vi "SWERVE_DRIVE_MODULE_ACT.vi"(8 "SwervePosInDeadband":bool=TRUE, 9 "Swerve Sense":T2={"Speed"=0.0, "Angle"={"VALUE"=0.0, "COS"=1.0, "SIN"=0.0}} {"Angle"."SIN" format="%13.4f"; "Angle"."COS" format="%13.4f"; "Angle"."VALUE" format="%13.4f"}, 10 "Swerve Dmd":T2={"Speed"=0.0, "Angle"={"VALUE"=0.0, "COS"=1.0, "SIN"=0.0}} {"Angle"."SIN" format="%13.4f"; "Angle"."COS" format="%13.4f"; "Angle"."VALUE" format="%13.4f"}, 11 "Swerve Module TypDef":T4) -> (0 "SwerveOnTarget":bool, 1 "SwervePosError":dbl, 2 "Swerve Motor Dmd":dbl, 3 "Wheel Motor Dmd":dbl, 4 "WheelSpeedErr":dbl)   [LabVIEW 2019]
uses:
  SWERVE_DRIVE_MODULE_TYPDEF.ctl
  <vilib>/Rock Robotics/WPI/MotorControl/WPI_MotorControlDeviceRef.ctl
  <vilib>/Rock Robotics/WPI/MotorControl/WPI_MotorControlType.ctl
  <vilib>/Rock Robotics/SystemInterfaces/DIO/FPGA_DIOPWMChannel.ctl
  <vilib>/Rock Robotics/WPI/PWM/WPI_PWMDeadband.ctl
  <vilib>/Rock Robotics/SystemInterfaces/DIO/FPGA_DIOChannel.ctl
  <vilib>/Rock Robotics/WPI/Encoder/WPI_EncoderDevRef.ctl
  <vilib>/Rock Robotics/SystemInterfaces/Encoder/FPGA_EncoderIdx.ctl
  <vilib>/Rock Robotics/SystemInterfaces/Counter/FPGA_CounterCtrSystemIndex.ctl
  <vilib>/Rock Robotics/WPI/Encoder/WPI_EncoderType.ctl
  <vilib>/Rock Robotics/WPI/ThirdParty/JAS_Junk/TrajLib/TypeDef/SWERVE_DRIVE_MODULE_STATE.ctl
  <vilib>/Rock Robotics/WPI/ThirdParty/JAS_Junk/TrajLib/TypeDef/ROTATION2D.ctl
  SWERVE_MODULE_MOTOR_CO.ctl
  <vilib>/Rock Robotics/WPI/ThirdParty/JAS_Junk/TrajLib/SlewRateLimiter_New.vi
  <vilib>/Rock Robotics/WPI/ThirdParty/JAS_Junk/TrajLib/SlewRateLimiter_Reset.vi
  <vilib>/Rock Robotics/WPI/ThirdParty/JAS_Junk/TrajLib/SlewRateLimiter_Calculate.vi
  <vilib>/Rock Robotics/WPI/ThirdParty/JAS_Junk/TrajLib/SlewRateLimiter_SetRate.vi
  <vilib>/Rock Robotics/WPI/ThirdParty/JAS_Junk/TrajLib/Util_GetTime.vi
  <vilib>/addons/control/pid/pid.llb/PID (DBL).vi
  <vilib>/addons/control/pid/NI_PID_pid.lvlib
  Secret_Control_Library_Protected/Secret_Control_Library_Protected.lvlib
  <vilib>/Rock Robotics/WPI/ThirdParty/JAS_Junk/TrajLib/Trajectory_Library.lvlib
panel:
  in  "Speed PID":T1={"proportional gain (Kc)"=0.45, "integral time (Ti, min)"=0.008, "derivative time (Td, min)"=0.0} {"derivative time (Td, min)" format="%.3f"; "integral time (Ti, min)" format="%.3f"; "proportional gain (Kc)" format="%.3f"}
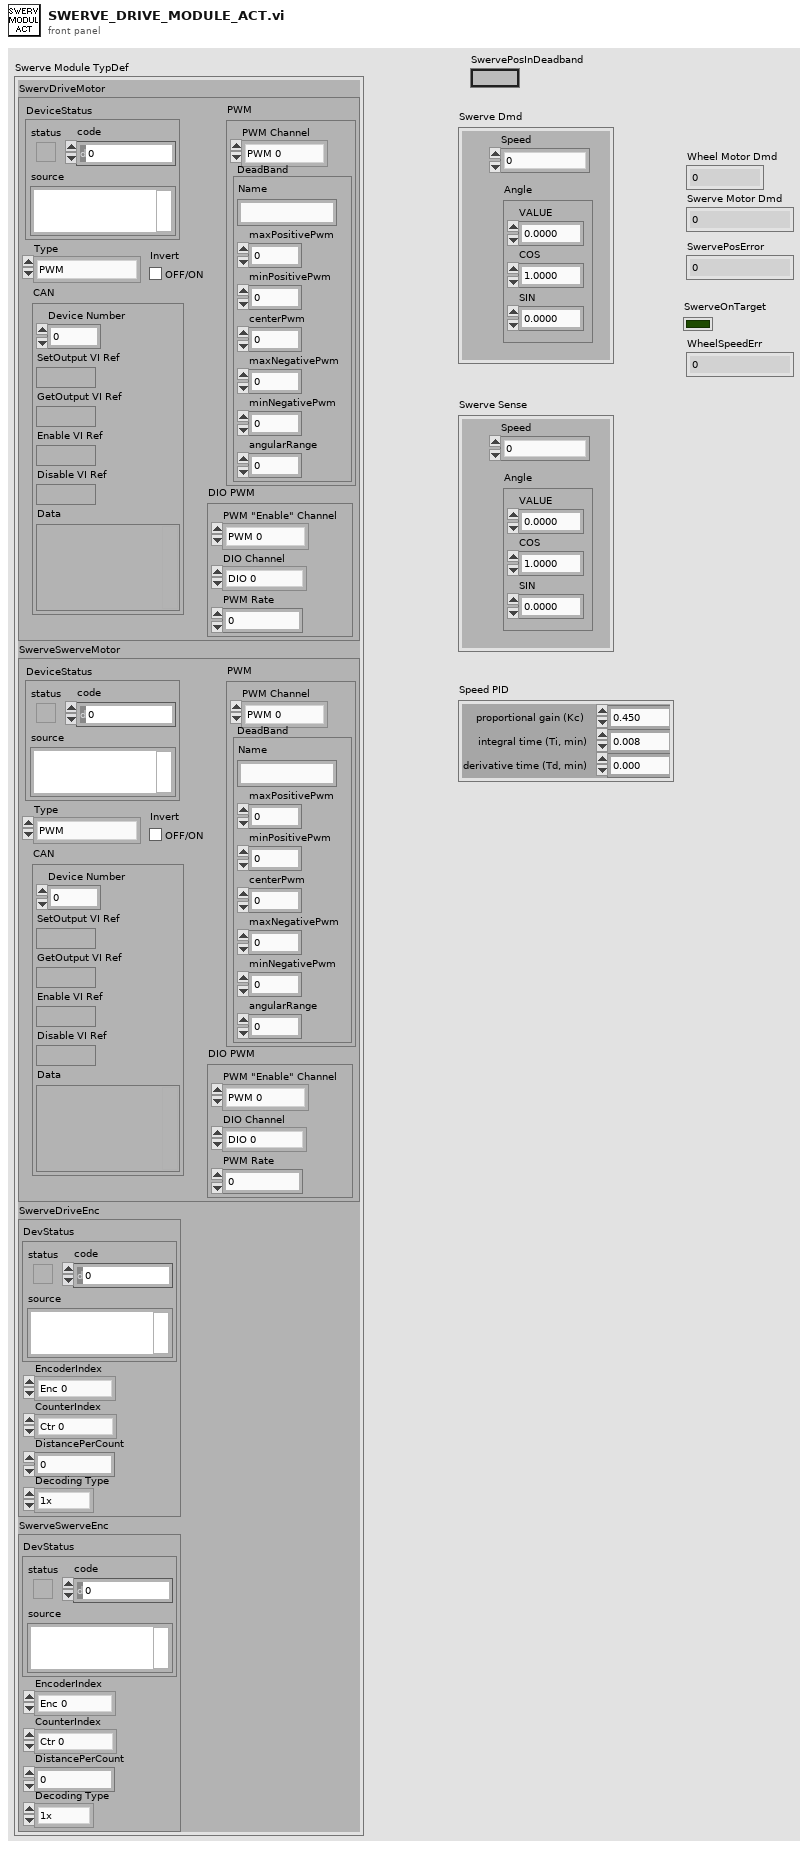
[diagram p1: front panel]
types:
  T1 = cluster{"proportional gain (Kc)":dbl, "integral time (Ti, min)":dbl, "derivative time (Td, min)":dbl}
  T2 = typedef "Trajectory_Library.lvlib/SWERVE_DRIVE_MODULE_STATE.ctl" = cluster{"Speed":dbl, "Angle":T3}
  T3 = typedef "Trajectory_Library.lvlib/ROTATION2D.ctl" = cluster{"VALUE":dbl, "COS":dbl, "SIN":dbl}
  T4 = typedef "SWERVE_DRIVE_MODULE_TYPDEF.ctl" = cluster{"SwervDriveMotor":T5, "SwerveSwerveMotor":T5, "SwerveDriveEnc":T10, "SwerveSwerveEnc":T10}
  T5 = typedef "WPI_MotorControlDeviceRef.ctl" = cluster{"DeviceStatus":errorcluster, "Type":T6, "PWM":cluster{"PWM Channel":T7, "DeadBand":T8}, "CAN":cluster{"Device Number":u8, "SetOutput VI Ref":variant, "GetOutput VI Ref":variant, "Enable VI Ref":variant, "Disable VI Ref":variant, "Data":variant}, "Invert":bool, "DIO PWM":cluster{"PWM \"Enable\" Channel":T7, "DIOChannel":T9, "PWM Rate":dbl}}
  T6 = typedef "WPI_MotorControlType.ctl" = enum16{"PWM", "CAN", "DIO PWM"}
  T7 = typedef "FPGA_DIOPWMChannel.ctl" = enum8{"PWM 0", "PWM 1", "PWM 2", "PWM 3", "PWM 4", "PWM 5", "PWM 6", "PWM 7", "PWM 8", "PWM 9", "PWM MXP 0", "PWM MXP 1", "PWM MXP 2", "PWM MXP 3", "PWM MXP 4", "PWM MXP 5", "PWM MXP 6", "PWM MXP 7", "PWM MXP 8", "PWM MXP 9", "Invalid"}
  T8 = typedef "WPI_PWMDeadband.ctl" = cluster{"Name":string, "maxPositivePwm":i32, "minPositivePwm":i32, "centerPwm":i32, "maxNegativePwm":i32, "minNegativePwm":i32, "angularRange":u16}
  T9 = typedef "FPGA_DIOChannel.ctl" = enum8{"DIO 0", "DIO 1", "DIO 2", "DIO 3", "DIO 4", "DIO 5", "DIO 6", "DIO 7", "DIO 8", "DIO 9", "DIO MXP 0", "DIO MXP 1", "DIO MXP 2", "DIO MXP 3", "DIO MXP 4", "DIO MXP 5", "DIO MXP 6", "DIO MXP 7", "DIO MXP 8", "DIO MXP 9", "DIO MXP 10", "DIO MXP 11", "DIO MXP 12", "DIO MXP 13", "DIO MXP 14", "DIO MXP 15", "SPI Port CS1", "SPI Port CS2", "SPI Port CS3", "SPI Port MISO", "SPI Port MOSI", "Invalid"}
  T10 = typedef "WPI_EncoderDevRef.ctl" = cluster{"DevStatus":errorcluster, "EncoderIndex":T11, "CounterIndex":T12, "DistancePerCount":dbl, "Decoding Type":T13}
  T11 = typedef "FPGA_EncoderIdx.ctl" = enum8{"Enc 0", "Enc 1", "Enc 2", "Enc 3", "Enc 4", "Enc 5", "Enc 6", "Enc 7", "Invalid"}
  T12 = typedef "FPGA_CounterCtrSystemIndex.ctl" = enum8{"Ctr 0", "Ctr 1", "Ctr 2", "Ctr 3", "Ctr 4", "Ctr 5", "Ctr 6", "Ctr 7", "Invalid"}
  T13 = typedef "WPI_EncoderType.ctl" = enum16{"1x", "2x", "4x"}
  T14 = typedef "SWERVE_MODULE_MOTOR_CO.ctl" = cluster{"WheelMotorDmd":dbl, "SwerveMotorDmd":dbl}
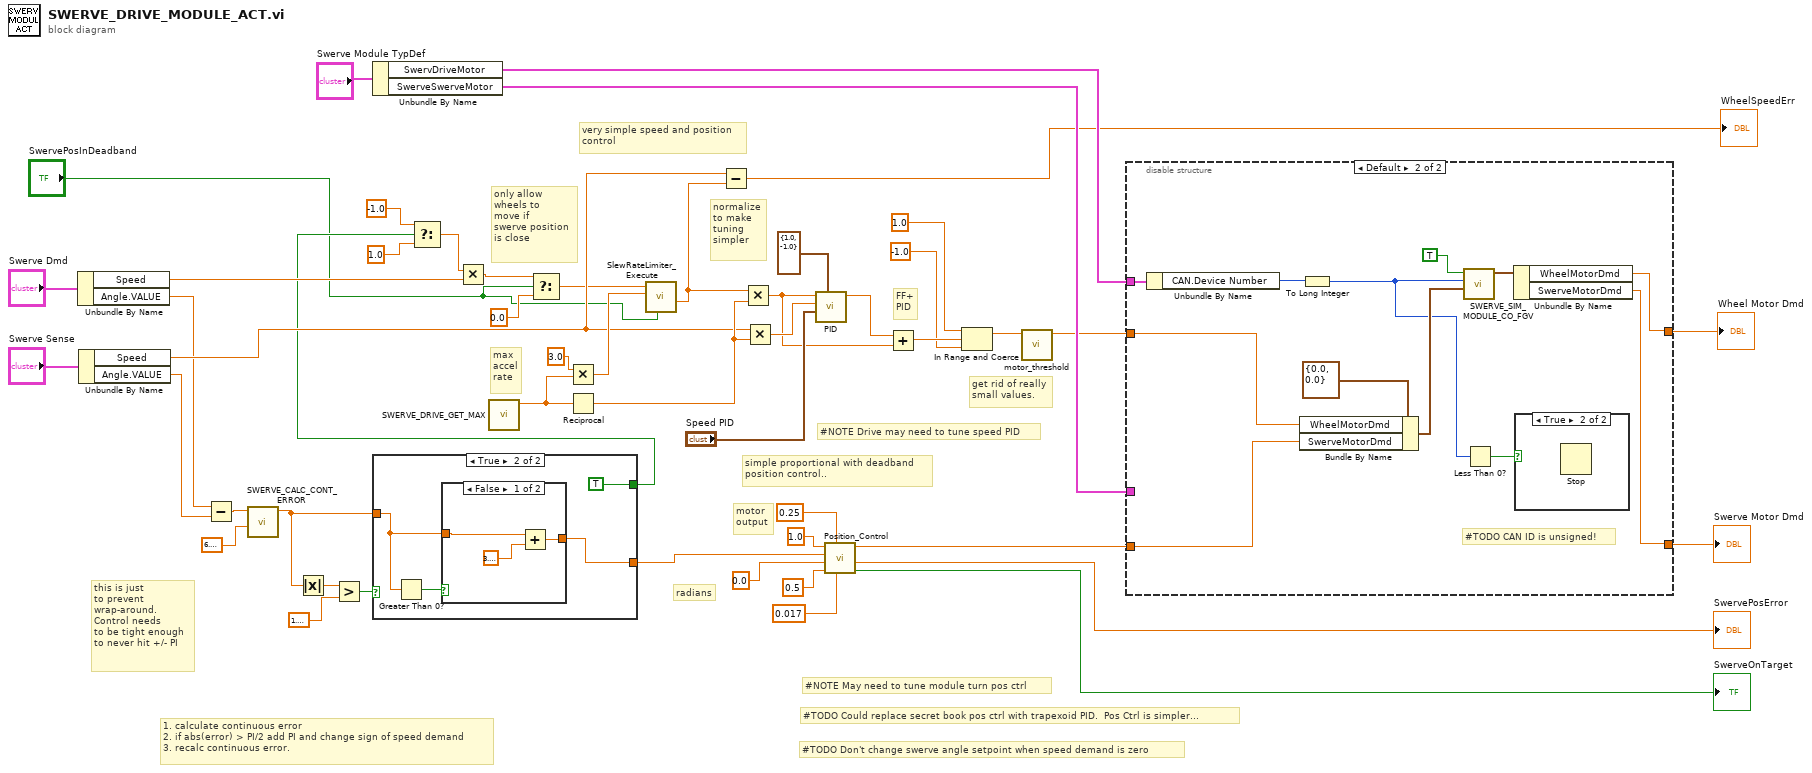
[diagram p0: block diagram]
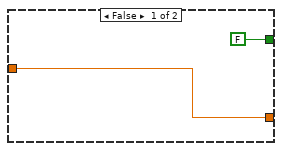
[diagram p2: hidden frame]
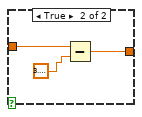
[diagram p3: hidden frame]
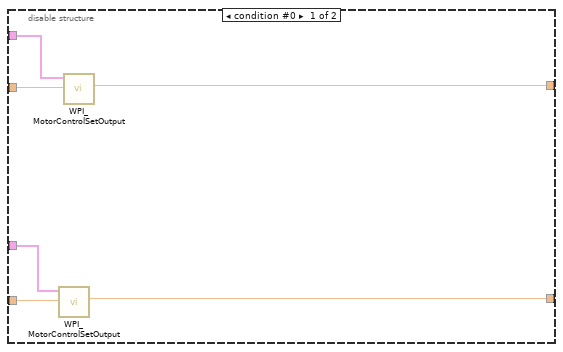
[diagram p4: hidden frame]
diagram:
  # "only allow\nwheels to \nmove if \nswerve position\nis close"
  # "#TODO Don't change swerve angle setpoint when speed demand is zero"
  # "1. calculate continuous error\n2. if abs(error) > PI/2 add PI and change sign of speed demand\n3. recalc continuous error."
  # "radians"
  # "#NOTE Drive may need to tune speed PID"
  # "#TODO Could replace secret book pos ctrl with trapexoid PID.  Pos Ctrl is simpler..."
  # "#NOTE May need to tune module turn pos ctrl"
  # "simple proportional with deadband\nposition control.."
  # "motor\noutput"
  # "this is just\nto prevent\nwrap-around.\nControl needs\nto be tight enough\nto never hit +/- PI"
  # "very simple speed and position\ncontrol"
  # "get rid of really\nsmall values."
  # "max\naccel\nrate"
  # "normalize\nto make\ntuning\nsimpler"
  # "FF+\nPID"
  n1 = Unbundle By Name("Swerve Dmd") -> ("Speed"=w23:dbl, "Angle.VALUE"=w7:dbl)
  n2 = Unbundle By Name("Swerve Sense") -> ("Speed"=w18:dbl, "Angle.VALUE"=w8:dbl)
  n3 = Subtract(x=w7, y=w8) -> (x-y=w15:dbl)
  n4 = call "SWERVE_CALC_CONT_ERROR.vi"("ErrorRange"=6.283185307179586, "Error"=w15) -> ("Continuous Error"=w9:dbl)  [unwired: 9 in]
  n5 = Absolute Value(x=w9) -> (abs(x)=w13:dbl)
  n6 = Greater?(x=w13, y=1.5707963267948966) -> (0:w11:bool)
  n7 = Unbundle By Name("Swerve Module TypDef") -> ("SwervDriveMotor"=w28:T5, "SwerveSwerveMotor"=w30:T5)
  n8 = case shown="True" w11 {
    tunnel: [FALSE TRUE] -> w10
    tunnel: [w51 w53] -> w5
    tunnel: w9 -> [w51 w54]
    frame False {
    }
    frame True {
      n9 = Greater Than 0?(x=w54) -> (x > 0?=w55:bool)
      n10 = case shown="False" w55 {
        tunnel: w54 -> [w58 w61]
        tunnel: [w59 w60] -> w53
        frame False {
          n11 = Add(x=w58, y=3.141592653589793) -> (x+y=w59:dbl)
        }
        frame True {
          n12 = Subtract(x=w61, y=3.141592653589793) -> (x-y=w60:dbl)
        }
      }
    }
  }
  n13 = Select(t=-1.0, s=w10, f=1.0) -> (s? t:f=w22:dbl)
  n14 = Multiply(x=w22, y=w23) -> (x*y=w3:dbl)
  n15 = call "SWERVE_DRIVE_GET_MAX.vi"() -> ("Max Wheel Vel (Meter/Sec)"=w38:dbl)  [unwired: 10 in, 1 out]
  n16 = Select(t=w3, s="SwervePosInDeadband", f=0.0) -> (s? t:f=w4:dbl)
  n17 = Multiply(x=3.0, y=w38) -> (x*y=w21:dbl)
  n18 = Reciprocal(x=w38) -> (1/x=w40:dbl)
  n19 = call <vilib>:"SlewRateLimiter_Execute.vi"("Enable"="SwervePosInDeadband", "PositiveRate"=w21, "Input"=w4) -> ("Output"=w17:dbl)  [unwired: 7 in, 1 out]
  n20 = Subtract(x=w18, y=w17) -> (x-y=→"WheelSpeedErr":dbl)
  n21 = Multiply(x=w17, y=w40) -> (x*y=w42:dbl)
  n22 = Multiply(x=w18, y=w40) -> (x*y=w43:dbl)
  n23 = call-poly <vilib>:"PID.vi"("output range"=cluster{"output high":dbl, "output low":dbl} {"output high"=1.0, "output low"=-1.0}, "PID gains"="Speed PID", "process variable"=w43, "setpoint"=w42) -> ("output"=w49:dbl)  [unwired: 6 in, 1 out]
  n24 = call "Position_Control.vi"("ErrDeadband"=0.017, "MinOutput"=0.25, "ErrThreshold"=0.5, "CurrentPosition"=0.0 ("TargetPosition"), "TargetPosition"=w5, "MaxOutput"=1.0) -> ("OnTarget"=→"SwerveOnTarget":bool, "PositionError"=→"SwervePosError":dbl, "Output"=w31:dbl)  [unwired: 3 in]
  n25 = Add(x=w49, y=w42) -> (x+y=w48:dbl)
  n26 = In Range and Coerce(upper limit=1.0, x=w48, lower limit=-1.0) -> (coerced(x)=w39:dbl)  [unwired: 1 out]
  n27 = call "motor_threshold.vi"("motor in"=w39) -> ("motor out"=w29:dbl)  [unwired: 10 in]
  n28 = disable-structure shown="Default" {
    disable-tunnel: w31 -> [w68 w76]
    disable-tunnel: w30 -> [w67 _]
    disable-tunnel: w29 -> [w66 w77]
    disable-tunnel: w28 -> [w65 w80]
    disable-tunnel: [w64 w72] -> w27
    disable-tunnel: [w63 w71] -> w26
    frame condition #0 {
      n29 = call <vilib>:"WPI_MotorControlSetOutput.vi"("Output"=w68, "MotorControlDevRef"=w67) -> ("Motor Output"=w63:dbl)  [unwired: 7 in, 2 out]
      n30 = call <vilib>:"WPI_MotorControlSetOutput.vi"("Output"=w66, "MotorControlDevRef"=w65) -> ("Motor Output"=w64:dbl)  [unwired: 7 in, 2 out]
    }
    frame condition #1 (active) {
      # "#TODO CAN ID is unsigned!"
      n31 = Unbundle By Name(w80) -> ("CAN.Device Number"=w70:u8)
      n32 = Bundle By Name(cluster=T14 {"WheelMotorDmd"=0.0, "SwerveMotorDmd"=0.0} ("SwerveModuleMotorDmd"), "WheelMotorDmd"=w77, "SwerveMotorDmd"=w76) -> (w75:T14)
      n33 = To Long Integer(number=w70) -> (32bit integer=w69:i32)
      n34 = call "SWERVE_SIM_MODULE_CO_FGV.vi"("in SwerveModuleMotorDmd"=w75, "Index"=w69, "WRITE"=TRUE) -> ("out SwerveModuleMotorDmd"=w73:T14)  [unwired: 8 in]
      n35 = Less Than 0?(x=w69) -> (x < 0?=w74:bool)
      n36 = Unbundle By Name(w73) -> ("WheelMotorDmd"=w72:dbl, "SwerveMotorDmd"=w71:dbl)
      n37 = case shown="True" w74 {
        frame False {
        }
        frame True {
          n38 = Stop() -> ()  [unwired: 1 in]
        }
      }
    }
  }
  "Wheel Motor Dmd" <- w27
  "Swerve Motor Dmd" <- w26
